vi "USRManager.vi"(3 "error in (no error)":errorcluster caption="错误输入（无错误）", 4 "Input":T1, 5 "ref_in":variant) -> (0 "error out":errorcluster caption="错误输出", 1 "Output":T1, 2 "ref_out":variant)   [LabVIEW 2012]
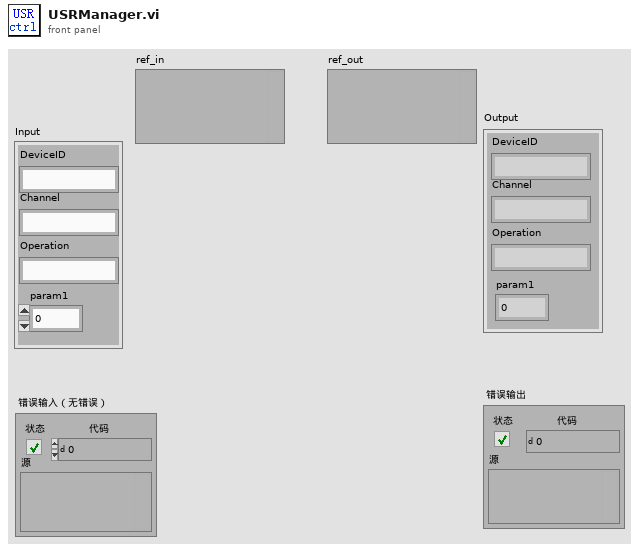
[diagram p1: front panel]
types:
  T1 = cluster{"DeviceID":string, "Channel":string, "param1":dbl, "Operation":string}
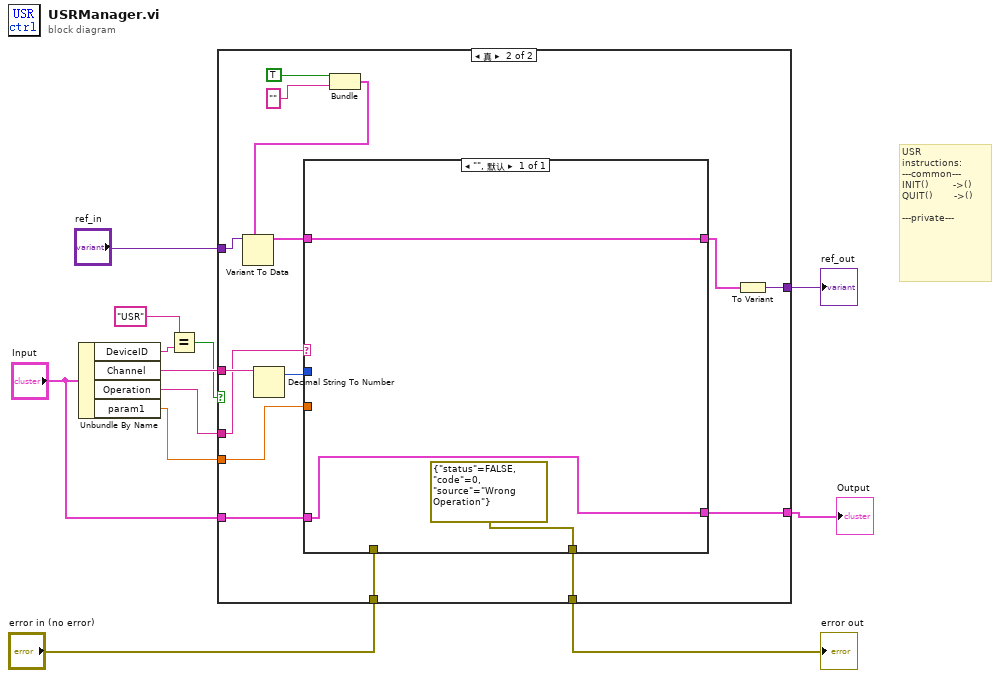
[diagram p0: block diagram]
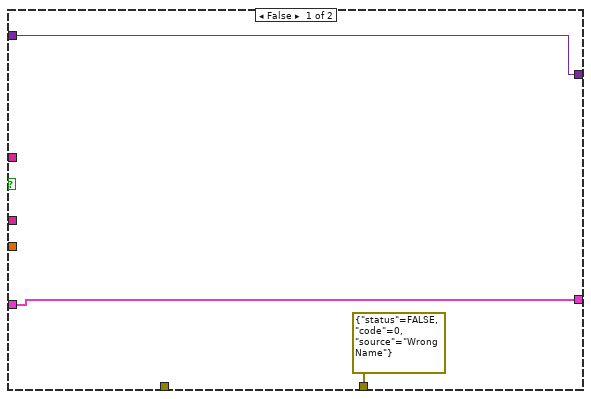
[diagram p2: hidden frame]
diagram:
  # "USR\ninstructions:\n---common---\nINIT()        ->()\nQUIT()       ->()\n\n---private---"
  n1 = Unbundle By Name("Input") -> ("DeviceID"=w12:string, "Channel"=w10:string, "Operation"=w9:string, "param1"=w8:dbl)
  n2 = Equal?(x="USR", y=w12) -> (x = y?=w3:bool)
  n3 = case shown="真" w3 {
    tunnel: w10 -> [_ w30]
    tunnel: w9 -> [_ w29]
    tunnel: w8 -> [_ w28]
    tunnel: "error in (no error)" -> [_ w27]
    tunnel: [errorcluster {"status"=FALSE, "code"=0, "source"="Wrong Name"} ("error out") w26] -> w6
    tunnel: [w15 w25] -> w5
    tunnel: "ref_in" -> [w13 w21]
    tunnel: "Input" -> [w15 w24]
    tunnel: [w13 w22] -> w2
    frame False {
    }
    frame True {
      n4 = Decimal String To Number(string=w30) -> (offset past number=w23:i32)  [unwired: 2 in, 1 out]
      n5 = Bundle(TRUE, "") -> (w20:cluster{bool, string})  [unwired: 1 in]
      n6 = Variant To Data(type=w20, Variant=w21) -> (data=w18:cluster{bool, string})  [unwired: 1 in, 1 out]
      n7 = case shown="\"\", 默认" w29 {
        tunnel: w28 -> [_]
        tunnel: w27 -> [_]
        tunnel: [errorcluster {"status"=FALSE, "code"=0, "source"="Wrong Operation"} ("error out")] -> w26
        tunnel: [w32] -> w25
        tunnel: w24 -> [w32]
        tunnel: w23 -> [_]
        tunnel: w18 -> [w31]
        tunnel: [w31] -> w16
        frame "", Default {
        }
      }
      n8 = To Variant(anything=w16) -> (Variant=w22:variant)
    }
  }
  "Output" <- w5
  "error out" <- w6
  "ref_out" <- w2
